vi "GDSError_VariantLog.vi"(2 "cases":T1=enum."AddError", 3 "VariantError":variant, 5 "error in (no error)":errorcluster, 9 "DeleteWhenRead":bool) -> (16 "ErrorArray":variant[](array[variant]), 19 "error out":errorcluster)   [LabVIEW 2020]
uses:
  GDSError_LogCases.ctl
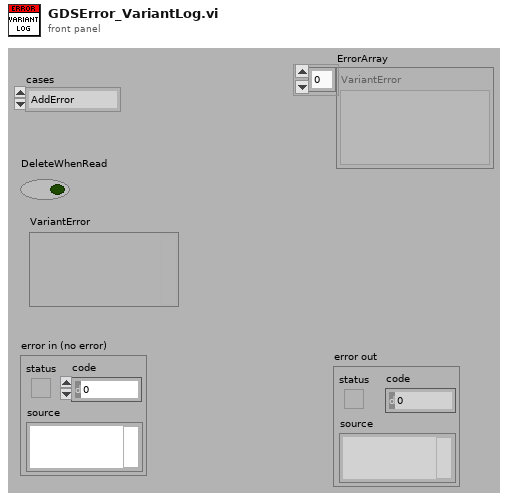
[diagram p1: front panel]
types:
  T1 = typedef "GDSError_LogCases.ctl" = enum16{"Init", "AddError", "ReadFirstError", "ReadLatestError", "ReadAllErrors", "ClearError", "ClearAllErrors"}
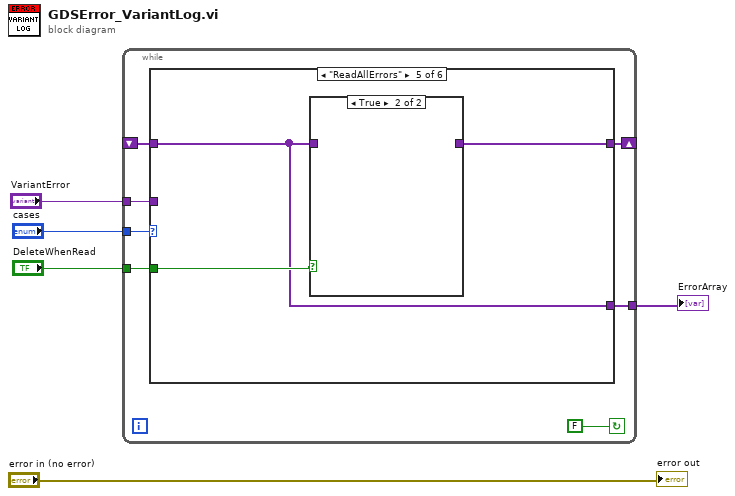
[diagram p0: block diagram]
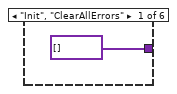
[diagram p2: hidden frame]
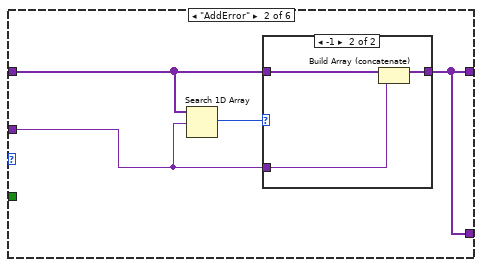
[diagram p3: hidden frame]
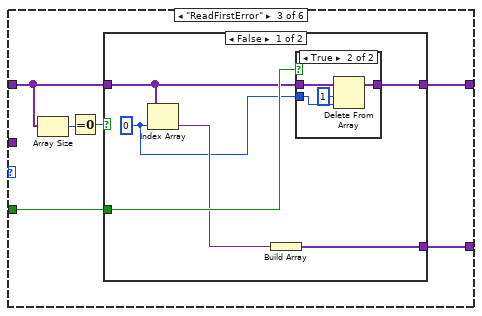
[diagram p5: hidden frame]
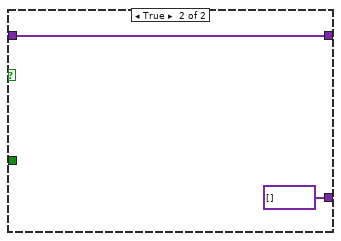
[diagram p7: hidden frame]
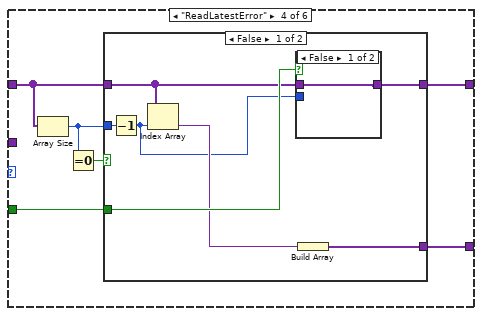
[diagram p8: hidden frame]
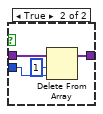
[diagram p9: hidden frame]
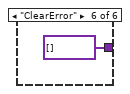
[diagram p12: hidden frame]
diagram:
  n1 = while {
    shift-right: [w10] -> _
    shift-left: _ -> [w9]
    tunnel: "cases" -> [w11]
    tunnel: [w8] -> w1
    tunnel: "DeleteWhenRead" -> [w7]
    tunnel: "VariantError" -> [w6]
    stop <- FALSE continue-if-true
    n2 = case shown="\"ReadAllErrors\"" w11 {
      tunnel: [variant[] [] ("ErrorArray") w14 w27 w46 w60 variant[] [] ("ErrorArray")] -> w10
      tunnel: w9 -> [_ w16 w25 w44 w61 _]
      tunnel: [_ w14 w24 w43 w61 _] -> w8
      tunnel: w7 -> [_ _ w26 w45 w62 _]
      tunnel: w6 -> [_ w15 _ _ _ _]
      frame "Init", "ClearAllErrors" {
      }
      frame "AddError" {
        n3 = Search 1D Array(1D array=w16, element=w15) -> (index of element=w17:i32)  [unwired: 1 in]
        n4 = case shown="-1" w17 {
          tunnel: [w18 w21] -> w14
          tunnel: w16 -> [w18 w20]
          tunnel: w15 -> [_ w19]
          frame 0.., Default {
            # "Error already\nadded"
          }
          frame -1 {
            n5 = Build Array (concatenate)(w20, w19) -> (w21:variant[])
          }
        }
      }
      frame "ReadFirstError" {
        n6 = Array Size(array=w25) -> (size(s)=w22:i32)
        n7 = Equal To 0?(x=w22) -> (x = 0?=w23:bool)
        n8 = case shown="False" w23 {
          tunnel: [w33 w40] -> w27
          tunnel: w26 -> [w32 _]
          tunnel: w25 -> [w31 w40]
          tunnel: [w28 variant[] []] -> w24
          frame False {
            w29 = 0
            n9 = Index Array(array=w31, index=w29) -> (element=w30:variant)
            n10 = Build Array(w30) -> (w28:variant[])
            n11 = case shown="True" w32 {
              tunnel: [w34 w36] -> w33
              tunnel: w31 -> [w34 w38]
              tunnel: w29 -> [_ w37]
              frame False {
              }
              frame True {
                n12 = Delete From Array(array=w38, length=1, index=w37) -> (array with subset deleted=w36:variant[])  [unwired: 1 out]
              }
            }
          }
          frame True {
          }
        }
      }
      frame "ReadLatestError" {
        n13 = Array Size(array=w44) -> (size(s)=w42:i32)
        n14 = Equal To 0?(x=w42) -> (x = 0?=w41:bool)
        n15 = case shown="False" w41 {
          tunnel: [w53 w59] -> w46
          tunnel: w45 -> [w52 _]
          tunnel: w44 -> [w51 w59]
          tunnel: [w47 _] -> w43
          tunnel: w42 -> [w48 _]
          frame False {
            n16 = Decrement(x=w48) -> (x-1=w49:i32)
            n17 = Index Array(array=w51, index=w49) -> (element=w50:variant)
            n18 = case shown="False" w52 {
              tunnel: [w54 w56] -> w53
              tunnel: w51 -> [w54 w58]
              tunnel: w49 -> [_ w57]
              frame False {
              }
              frame True {
                n19 = Delete From Array(array=w58, length=1, index=w57) -> (array with subset deleted=w56:variant[])  [unwired: 1 out]
              }
            }
            n20 = Build Array(w50) -> (w47:variant[])
          }
          frame True {
          }
        }
      }
      frame "ReadAllErrors" {
        n21 = case shown="True" w62 {
          tunnel: w61 -> [w63 _]
          tunnel: [w63 _] -> w60
          frame False {
          }
          frame True {
          }
        }
      }
      frame "ClearError" {
      }
    }
  }
  "ErrorArray" <- w1
  "error out" <- "error in (no error)"
